vi "Get Node Attribute Value.vi"(9 "Default Value":string, 10 "Attribute Name":string, 11 "Refnum in":refnum<k20>) -> (3 "Value":string)   [LabVIEW 2025]
uses:
  <resource>/objmgr/DOMUserDefRef.rc
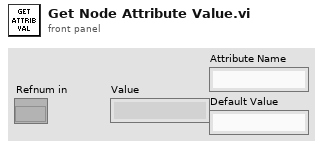
[diagram p1: front panel]
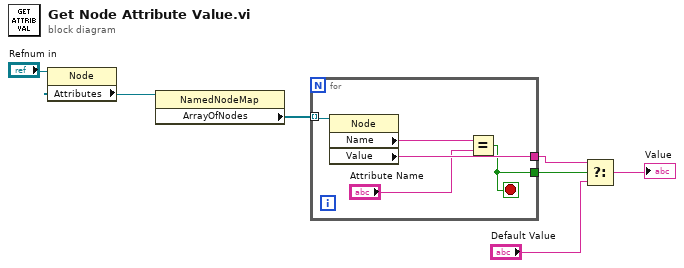
[diagram p0: block diagram]
diagram:
  n1 = property class="Node"(reference="Refnum in") -> ("Attributes"=w6:refnum<k20>)  [unwired: 1 in, 2 out]
  n2 = property class="NamedNodeMap"(reference=w6) -> ("ArrayOfNodes"=w7:refnum<k20>[])  [unwired: 1 in, 2 out]
  n3 = for {
    tunnel: w7 -> [w12] mode=indexing
    tunnel: [w10] -> w3
    tunnel: [w8] -> w4
    stop <- w8 stop-if-true
    n4 = property class="Node"(reference=w12) -> ("Name"=w11:string, "Value"=w10:string)  [unwired: 1 in, 2 out]
    n5 = Equal?(x=w11, y="Attribute Name") -> (x = y?=w8:bool)
  }
  n6 = Select(t=w3, s=w4, f="Default Value") -> (s? t:f=→"Value":string)
